vi "Actor Core.vi"(8 "error in":errorcluster, 11 "Controller in":refnum<class "Controller.lvclass">) -> (0 "error out":errorcluster, 3 "Actor out":refnum<class "Actor.lvclass">)   [LabVIEW 2014, in "Controller.lvclass"]
doc: "(<B>Filename</B>: Actor Framework.lvlib:Actor.lvclass:Actor Core.vi)\n\nReceives messages to the actor, reacts to them, and initiates any error handling that may shut the actor down.\n\nDescendant classes may override this VI to append parallel tasks for the actor to complete while it handles messages. Overrides use the Call Parent Method node."
uses:
  Controller.lvclass
  <vilib>/ActorFramework/Actor/Actor.lvclass
  Generic Instrument/Generic Instrument.lvclass
  <vilib>/ActorFramework/Message Enqueuer/Message Enqueuer.lvclass
  SetUp VIs/Instrument Finder/Instrument Finder.lvclass
  <vilib>/ActorFramework/Actor/Actor.lvclass/Actor.ctl
  <vilib>/ActorFramework/Message Enqueuer/Message Enqueuer.lvclass/Message Enqueuer.ctl
  Display Panel/Display Panel V3/Display Panel V3.lvclass
  Display Panel/Display Panel V3 Messages/Write String from Control Msg/Write String from Control Msg.lvclass/Write String from Control Msg.ctl
  Subpanel Inserter Messages/Insert Into Subpanel Msg/Insert Into Subpanel Msg.lvclass/Insert Into Subpanel Msg.ctl
  <vilib>/ActorFramework/Stop Msg/Stop Msg.lvclass/Stop Msg.ctl
  <vilib>/ActorFramework/Message Enqueuer/Init from Existing Queue.vi
  <vilib>/ActorFramework/Message Enqueuer/Enqueue.vi
  <vilib>/ActorFramework/Message Enqueuer/Enqueue Critical.vi
  <vilib>/ActorFramework/Message Priority Queue/Priority Enqueue.vi
  Display Panel/Display Panel V3 Messages/Write String from Control Msg/Write String from Control Msg.lvclass
  Subpanel Inserter Messages/Insert Into Subpanel Msg/Insert Into Subpanel Msg.lvclass
  Subpanel Inserter Messages/Send Stop Event Msg/Send Stop Event Msg.lvclass
  <vilib>/ActorFramework/Stop Msg/Stop Msg.lvclass
  <vilib>/MGI/Monitored Actor/Actor/Monitored Actor.lvclass
panel:
  out "stop i loop":i32
  out "Display Addresses":refnum<class "Message Enqueuer.lvclass">[](array[class])
  out "Instrument addresses":refnum<class "Message Enqueuer.lvclass">[](array[class])
  in  "OK Button":bool
  in  "Next Button":bool
  in  "Previous Button":bool
  out "Instrument finder done?":bool
  out "i":i32
  out "Array of Instruments":refnum<class "Generic Instrument.lvclass">[](array[class])
  in  "Stop Button":bool
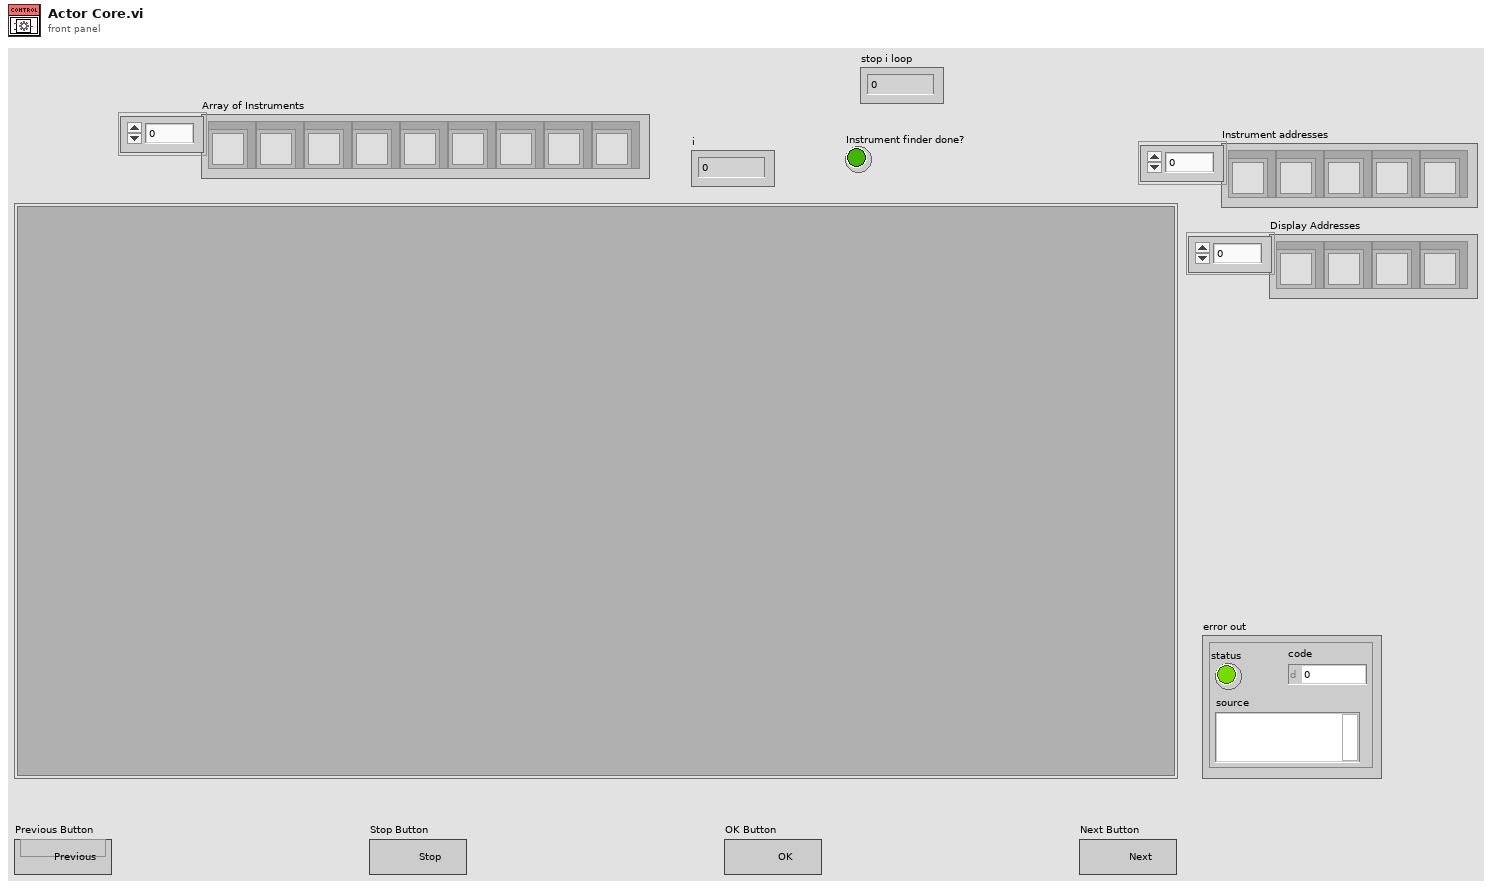
[diagram p1: front panel]
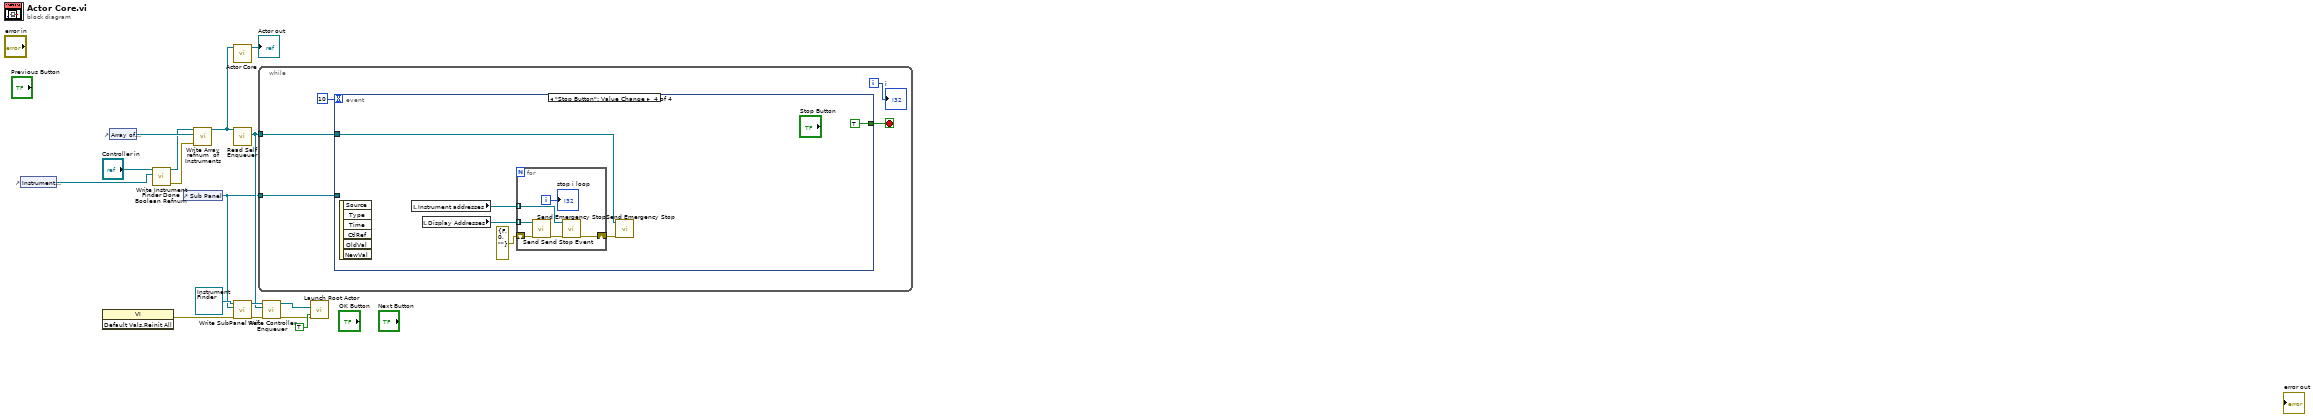
[diagram p0: block diagram]
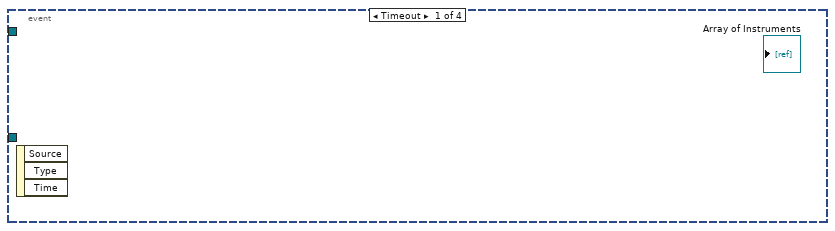
[diagram p2: hidden frame]
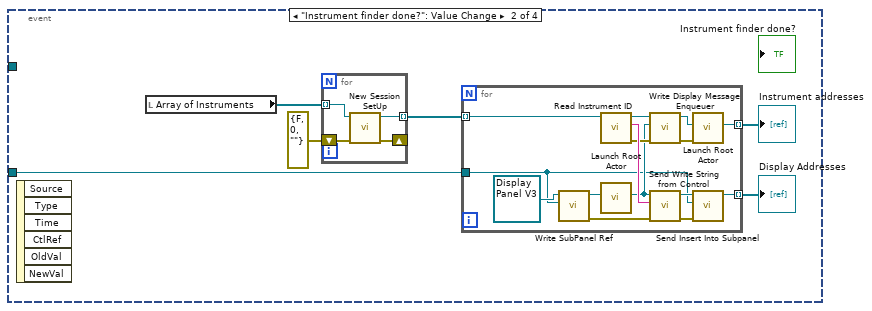
[diagram p3: hidden frame]
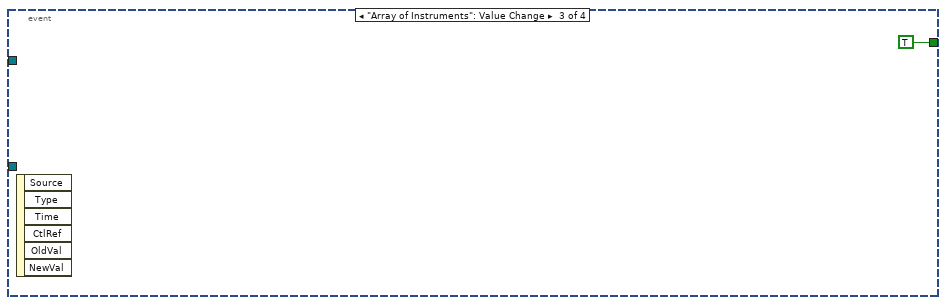
[diagram p4: hidden frame]
diagram:
  n1 = control-ref of="Instrument finder done?"() -> (w2:refnum<vi>)
  n2 = invoke class="VI" method="Default Vals.Reinit All"() -> (error out=w14:errorcluster)  [unwired: 3 in, 2 out]
  n3 = control-ref of="Array of Instruments"() -> (w7:refnum<vi>)
  n4 = call-dynamic "Write Instrument Finder Done Boolean Refnum.vi"("Instrument Finder Done Boolean Refnum"=w2, "Controller in"="Controller in") -> ("error out"=w3:errorcluster, "Controller out"=w4:refnum<class "Controller.lvclass">)  [unwired: 8 in]
  n5 = control-ref of="Sub Panel"() -> (w1:refnum<vi>)
  n6 = call-dynamic "Write Array refnum  of Instruments.vi"("error in (no error)"=w3, "Array refnum  of Instruments"=w7, "Controller in"=w4) -> ("Controller out"=w6:refnum<class "Controller.lvclass">)  [unwired: 7 in, 1 out]
  n7 = call-parent "Actor Core.vi"("Actor in"=w6) -> ("Actor out"=→"Actor out":refnum<class "Actor.lvclass">)  [unwired: 9 in, 1 out]
  n8 = call <vilib>:"Read Self Enqueuer.vi"("Actor"=w6) -> ("Self Enqueuer"=w8:refnum<class "Message Enqueuer.lvclass">)  [unwired: 10 in]
  n9 = call-dynamic "Write SubPanel Ref.vi"("error in (no error)"=w14, "SubPanel Ref"=w1, "Subpanel Inserter in"=refnum<class "Instrument Finder.lvclass"> refnum ("SetUp VIs.lvlib:Instrument Finder.lvclass")) -> ("error out"=w10:errorcluster, "Subpanel Inserter out"=w12:refnum<class "Instrument Finder.lvclass">)  [unwired: 7 in]
  n10 = while {
    tunnel: w8 -> [w19]
    tunnel: w1 -> [w17]
    i -> [w18]
    stop <- w20 stop-if-true
    n11 = event shown="[3] \"Stop Button\": Value Change" {
      selector: _ -> [_ _ _ _]
      dyn-events: _ -> [_ _ _ _]
      timeout: 10 -> [_ _ _ _]
      tunnel: [_ _ TRUE TRUE] -> w20
      tunnel: w19 -> [_ _ _ w52]
      tunnel: w17 -> [_ w23 _ _]
      event Timeout {
        n12 = event-data() -> ()  [unwired: 1 in, 3 out]
      }
      event "Instrument finder done?": Value Change {
        n13 = event-data() -> ()  [unwired: 1 in, 6 out]
        n14 = local read "Array of Instruments"() -> (w27:refnum<class "Generic Instrument.lvclass">[])
        n15 = for {
          tunnel: w27 -> [w46] mode=indexing
          shift-right: [w44] -> _
          shift-left: errorcluster {"status"=FALSE, "code"=0, "source"=""} ("error out") -> [w45]
          tunnel: [w43] -> w25 mode=indexing
          n16 = call-dynamic "New Session SetUp.vi"("error in (no error)"=w45, "Generic Instrument in"=w46) -> ("error out"=w44:errorcluster, "Generic Instrument out"=w43:refnum<class "Generic Instrument.lvclass">)  [unwired: 8 in]
        }
        n17 = for {
          tunnel: w25 -> [w39] mode=indexing
          tunnel: [w42] -> w24 mode=indexing
          tunnel: w23 -> [w29]
          tunnel: [w28] -> w22 mode=indexing
          n18 = call-dynamic "Write SubPanel Ref.vi"("SubPanel Ref"=w29, "Subpanel Inserter in"=refnum<class "Display Panel V3.lvclass"> refnum ("Display Panel.lvlib:Display Panel V3.lvclass")) -> ("error out"=w30:errorcluster, "Subpanel Inserter out"=w40:refnum<class "Display Panel V3.lvclass">)  [unwired: 8 in]
          n19 = call-dynamic "Read Instrument ID.vi"("Generic Instrument in"=w39) -> ("error out"=w35:errorcluster, "Instrument ID"=w38:string, "Generic Instrument out"=w37:refnum<class "Generic Instrument.lvclass">)  [unwired: 8 in]
          n20 = call <vilib>:"Launch Root Actor.vi"("Actor"=w40) -> ("Actor's Enqueuer"=w33:refnum<class "Message Enqueuer.lvclass">)  [unwired: 9 in, 1 out]
          n21 = call-dynamic "Write Display Message Enqueuer.vi"("error in (no error)"=w35, "Actor Framework.lvlib:Message Enqueuer"=w33, "Generic Instrument in"=w37) -> ("error out"=w34:errorcluster, "Generic Instrument out"=w36:refnum<class "Generic Instrument.lvclass">)  [unwired: 7 in]
          n22 = call "Send Write String from Control.vi"("error in (no error)"=w30, "String"=w38, "Message Enqueuer"=w33) -> ("error out"=w31:errorcluster, "Message Enqueuer out"=w32:refnum<class "Message Enqueuer.lvclass">)  [unwired: 7 in]
          n23 = call <vilib>:"Launch Root Actor.vi"("error in (no error)"=w34, "Actor"=w36) -> ("Actor's Enqueuer"=w42:refnum<class "Message Enqueuer.lvclass">)  [unwired: 8 in, 1 out]
          n24 = call "Send Insert Into Subpanel.vi"("error in (no error)"=w31, "SubPanel Ref"=w29, "Message Enqueuer"=w32) -> ("Message Enqueuer out"=w28:refnum<class "Message Enqueuer.lvclass">)  [unwired: 7 in, 1 out]
        }
        "Instrument addresses" <- w24
        "Display Addresses" <- w22
      }
      event "Array of Instruments": Value Change {
        n25 = event-data() -> ()  [unwired: 1 in, 6 out]
      }
      event "Stop Button": Value Change {
        n26 = event-data() -> ()  [unwired: 1 in, 6 out]
        n27 = local read "Instrument addresses"() -> (w48:refnum<class "Message Enqueuer.lvclass">[])
        n28 = local read "Display Addresses"() -> (w49:refnum<class "Message Enqueuer.lvclass">[])
        n29 = for {
          tunnel: w49 -> [w56] mode=indexing
          shift-right: [w59] -> w51
          shift-left: errorcluster {"status"=FALSE, "code"=0, "source"=""} ("error out") -> [w55]
          tunnel: w48 -> [w57] mode=indexing
          i -> [w58]
          n30 = call "Send Send Stop Event.vi"("error in (no error)"=w55, "Message Enqueuer"=w56) -> ("error out"=w54:errorcluster)  [unwired: 8 in, 1 out]
          n31 = call <vilib>:"Send Emergency Stop.vi"("error in (no error)"=w54, "Message Enqueuer"=w57) -> ("error out"=w59:errorcluster)  [unwired: 9 in]
          "stop i loop" <- w58
        }
        n32 = call <vilib>:"Send Emergency Stop.vi"("error in (no error)"=w51, "Message Enqueuer"=w52) -> ()  [unwired: 9 in, 1 out]
      }
    }
    "i" <- w18
  }
  n33 = call-dynamic "Write Controller Enqueuer.vi"("error in (no error)"=w10, "Actor Framework:Message Enqueuer"=w8, "Instrument Finder in"=w12) -> ("error out"=w9:errorcluster, "Instrument Finder out"=w11:refnum<class "Instrument Finder.lvclass">)  [unwired: 7 in]
  n34 = call <vilib>:"Launch Root Actor.vi"("Open Actor Core front panel? (F)"=TRUE, "error in (no error)"=w9, "Actor"=w11) -> ()  [unwired: 7 in, 2 out]
